vi "Get Message Queues.vi"(8 "error in (no error)":errorcluster) -> (0 "error out":errorcluster, 3 "AllMsgQueues QueueRef":T1, 5 "MsgQueues QueueRef":refnum<queue>)   [LabVIEW 2021, in "dcvmMessageQueue.lvlib"]
uses:
  dcvmMessageQueue.lvlib
  controls/Message Queues.ctl
  controls/Message Data.ctl
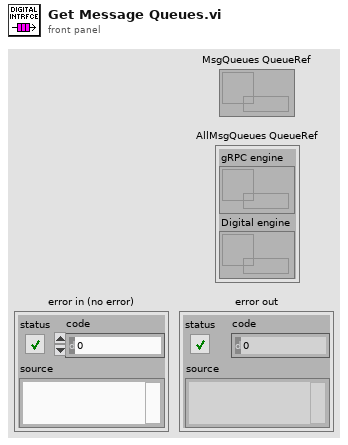
[diagram p1: front panel]
types:
  T1 = typedef "dcvmMessageQueue.lvlib/Message Queues.ctl" = cluster{"gRPC engine":refnum<queue>, "Digital engine":refnum<queue>}
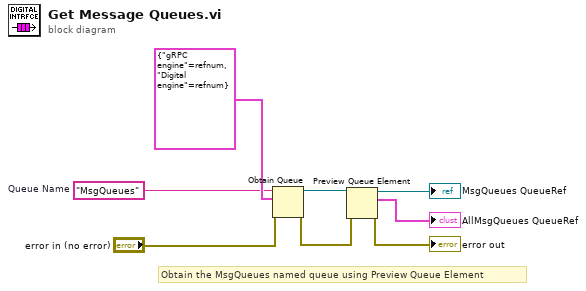
[diagram p0: block diagram]
diagram:
  w4 = "MsgQueues"  # Queue Name
  # "Obtain the MsgQueues named queue using Preview Queue Element"
  n1 = Obtain Queue(name (unnamed)=w4, element data type=T1 {"gRPC engine"=refnum, "Digital engine"=refnum} ("Message Queues"), error in (no error)="error in (no error)") -> (queue out=w7:refnum<queue>, error out=w3:errorcluster)  [unwired: 2 in, 1 out]
  n2 = Preview Queue Element(queue=w7, error in (no error)=w3) -> (queue out=→"MsgQueues QueueRef":refnum<queue>, element=→"AllMsgQueues QueueRef":T1, error out=→"error out":errorcluster)  [unwired: 1 in, 1 out]
